vi "LVDimInterface.dic_info_service_notifier.vi"(1 "serviceName":string, 2 "notifierRef":T2, 3 "timeout [s]":i32=10, 4 "serviceType":T1=4 items=["ONCE_ONLY"=1, "TIMED"=2, "MONITORED"=4], 5 "error in (no error)":errorcluster, 7 "stamped":bool=TRUE) -> (14 "callBackID":i32, 19 "error out":errorcluster)   [LabVIEW 2012, in "LVDimInterface.lvlib"]
doc: "Registers a notifier to a DIM service. The data received by DIM will be inserted as a new element to the notifier. If no longer used, a registered event should be unregistered using \"release service\".\n\nHistory: 16-DEC-2005, Dietrich Beck\n\nCopyright (C)\nGesellschaft für Schwerionenforschung, GSI\nPlanckstr. 1\n64291 Darmstadt\nGermany\n\nContact: D.Beck@gsi.de \n\nThis program is free software; you can redistribute it and/or modify it under the terms of the \nGNU General Public License as published by the Free Software Foundation; either version 2 of the license, or (at your option) any later version.\n\nThis program is distributed in the hope that it will be useful, but WITHOUT ANY WARRANTY; without even the implied warranty of MERCHANTABILITY or FITNESS FOR A PARTICULAR PURPOSE. See the GNU General License for more details (http://www.gnu.org).\n\nGesellschaft für Schwerionenforschung, GSI\nPlanckstr. 1, 64291 Darmstadt, Germany\nFor all questions and ideas contact D. Beck.\nLast update: 16-DEC-2005"
uses:
  LVDimInterface.lvlib
  LVDimInterface.notifier type.ctl
  LVDimInterface.dim service type.ctl
  bin/libDimWrapper.dll
  bin/libDimWrapper.so
  bin/libDimWrapperSPL.dll
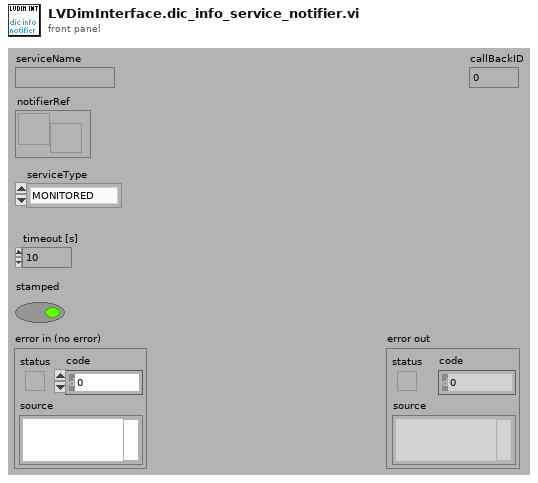
[diagram p1: front panel]
types:
  T1 = typedef "LVDimInterface.lvlib/LVDimInterface.dim service type.ctl" = u16
  T2 = typedef "LVDimInterface.lvlib/LVDimInterface.notifier type.ctl" = refnum<notifier>
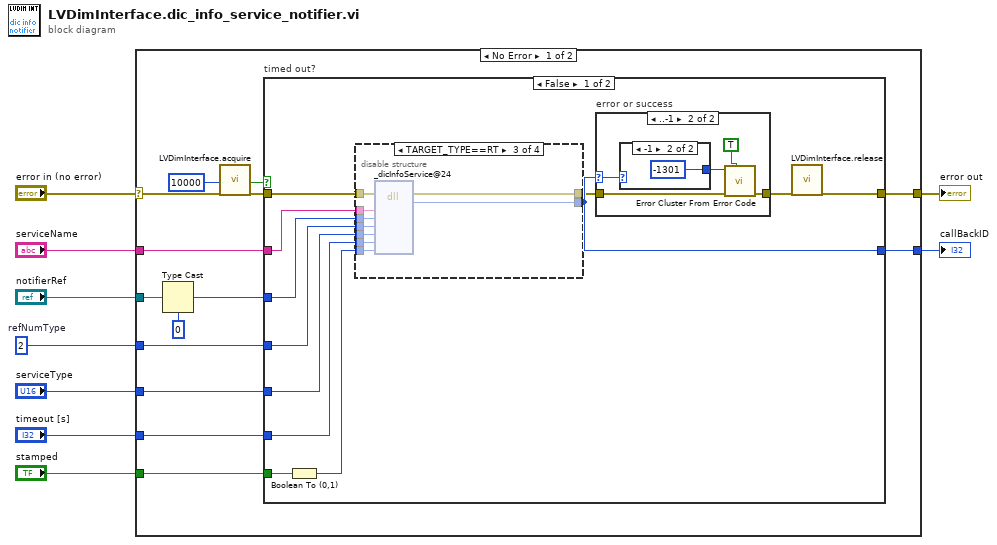
[diagram p0: block diagram]
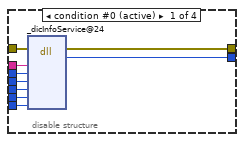
[diagram p2: hidden frame]
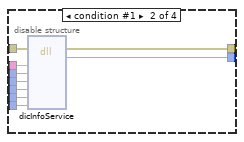
[diagram p3: hidden frame]
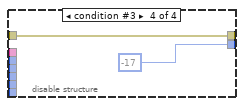
[diagram p4: hidden frame]
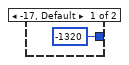
[diagram p6: hidden frame]
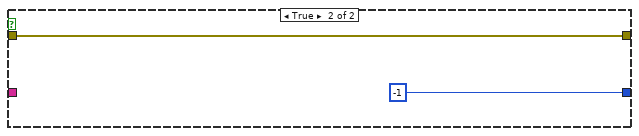
[diagram p7: hidden frame]
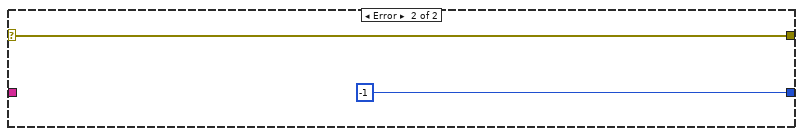
[diagram p8: hidden frame]
diagram:
  w7 = 2  # refNumType
  n1 = case shown="No Error" "error in (no error)" {
    selector: "error in (no error)" -> [w10 w76]
    tunnel: "serviceName" -> [w23 _]
    tunnel: "notifierRef" -> [w16 _]
    tunnel: w7 -> [w22 _]
    tunnel: "serviceType" -> [w21 _]
    tunnel: "timeout [s]" -> [w20 _]
    tunnel: [w18 -1 ("callBackID")] -> w4
    tunnel: [w19 w76] -> w2
    tunnel: "stamped" -> [w17 _]
    frame No Error {
      n2 = Type Cast(type=u32 0, x=w16) -> (*(type *) &x=w14:u32)
      n3 = call "LVDimInterface.acquire.vi"("ms timeout (10000)"=10000 ("ms timeout (-1)"), "error in (no error)"=w10) -> ("timed out"=w11:bool, "error out"=w13:errorcluster)  [unwired: 16 in]
      n4 = case "timed out?" shown="False" w11 {
        tunnel: w23 -> [w35 _]
        tunnel: w14 -> [w34 _]
        tunnel: w22 -> [w33 _]
        tunnel: w21 -> [w32 _]
        tunnel: w20 -> [w31 _]
        tunnel: [w24 w73] -> w19
        tunnel: [w30 -1 ("callBackID")] -> w18
        tunnel: w17 -> [w29 _]
        tunnel: w13 -> [w27 w73]
        frame False {
          n5 = Boolean To (0,1)(Boolean=w29) -> (0, 1=w28:i16)
          n6 = disable-structure "Conditional Disable Structure" shown="TARGET_TYPE==RT" {
            disable-tunnel: w35 -> [w44 w53 w62 _]
            disable-tunnel: w34 -> [w43 w52 w61 _]
            disable-tunnel: w33 -> [w42 w51 w60 _]
            disable-tunnel: w32 -> [w41 w50 w59 _]
            disable-tunnel: w31 -> [w40 w49 w58 _]
            disable-tunnel: [w39 w48 w57 -17 ("callBackID")] -> w30
            disable-tunnel: w28 -> [w38 w47 w56 _]
            disable-tunnel: w27 -> [w37 w46 w55 w63]
            disable-tunnel: [w36 w45 w54 w63] -> w26
            frame condition #0 (active) {
              n7 = dll-call lib="D:/DIMLVEvent LV2012/bin/libDimWrapper.dll" fn="_dicInfoService@24"(error in=w37, "serviceName"=w44, "refNum"=w43, "refNumType"=w42, "serviceType"=w41, "timeout"=w40, "stamped"=w38) -> (error out=w36:errorcluster, "callBackID"=w39:i32)  [unwired: 8 in, 1 out]
            }
            frame condition #1 {
              n8 = dll-call lib="D:/DIMLVEvent LV2012/bin/libDimWrapper.so" fn="dicInfoService" label="libDimWrapper.dll:_dicInfoService@24"(error in=w46, "serviceName"=w53, "refNum"=w52, "refNumType"=w51, "serviceType"=w50, "timeout"=w49, "stamped"=w47) -> (error out=w45:errorcluster, "callBackID"=w48:i32)  [unwired: 8 in, 1 out]
            }
            frame condition #2 {
              n9 = dll-call lib="D:/DIMLVEvent LV2012/bin/libDimWrapperSPL.dll" fn="_dicInfoService@24"(error in=w55, "serviceName"=w62, "refNum"=w61, "refNumType"=w60, "serviceType"=w59, "timeout"=w58, "stamped"=w56) -> (error out=w54:errorcluster, "callBackID"=w57:i32)  [unwired: 8 in, 1 out]
            }
            frame condition #3 {
            }
          }
          n10 = case "error or success" shown="..-1" w30 {
            selector: w30 -> [_ w70]
            tunnel: w26 -> [w65 w68]
            tunnel: [w65 w69] -> w25
            frame 0, Default {
            }
            frame ..-1 {
              n11 = case shown="-1" w70 {
                tunnel: [-1320 ("code") -1301 ("code")] -> w67
                frame -17, Default {
                }
                frame -1 {
                }
              }
              n12 = call <vilib>:"Error Cluster From Error Code.vi"("show call chain? (False)"=TRUE ("status"), "error in (no error)"=w68, "error code (0)"=w67) -> ("error out"=w69:errorcluster)  [unwired: 6 in]
            }
          }
          n13 = call "LVDimInterface.release.vi"("error in (no error)"=w25) -> ("error out"=w24:errorcluster)  [unwired: 18 in]
        }
        frame True {
        }
      }
    }
    frame Error {
    }
  }
  "callBackID" <- w4
  "error out" <- w2
